vi "Image_RGB888_to_RAW12_U8.vi"(7 "Bayer Pattern":T1, 8 "error in (no error)":errorcluster, 10 "Image Configuration":T2={"Width"=1920, "Height"=1080}, 11 "RGB Frame (U8)":u8[](array[numeric])) -> (0 "error out":errorcluster, 3 "RAW12 Frame (U8)":u8[](array[numeric]))   [LabVIEW 2020]
uses:
  ctl/Image_Configuration.ctl
  ctl/Image_RAW_Bayer_Pattern.ctl
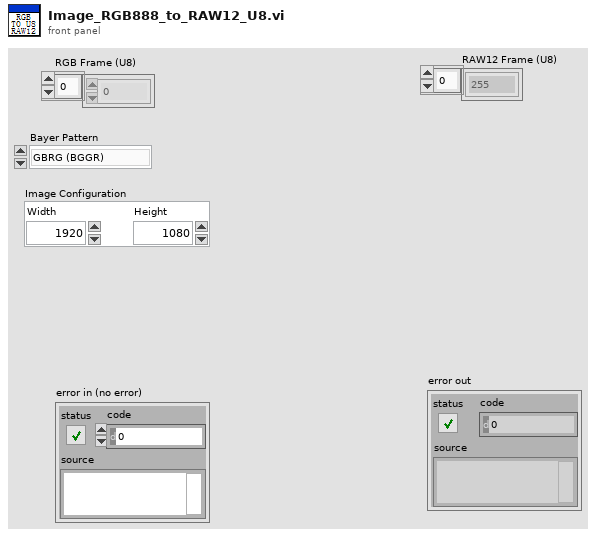
[diagram p1: front panel]
types:
  T1 = typedef "Image_RAW_Bayer_Pattern.ctl" = enum16{"GBRG (BGGR)", "GRBG (RGGB)", "BGGR (GBRG)", "RGGB (GRBG)", "CRBC (RCCB)"}
  T2 = typedef "Image_Configuration.ctl" = cluster{"Width":i32, "Height":i32}
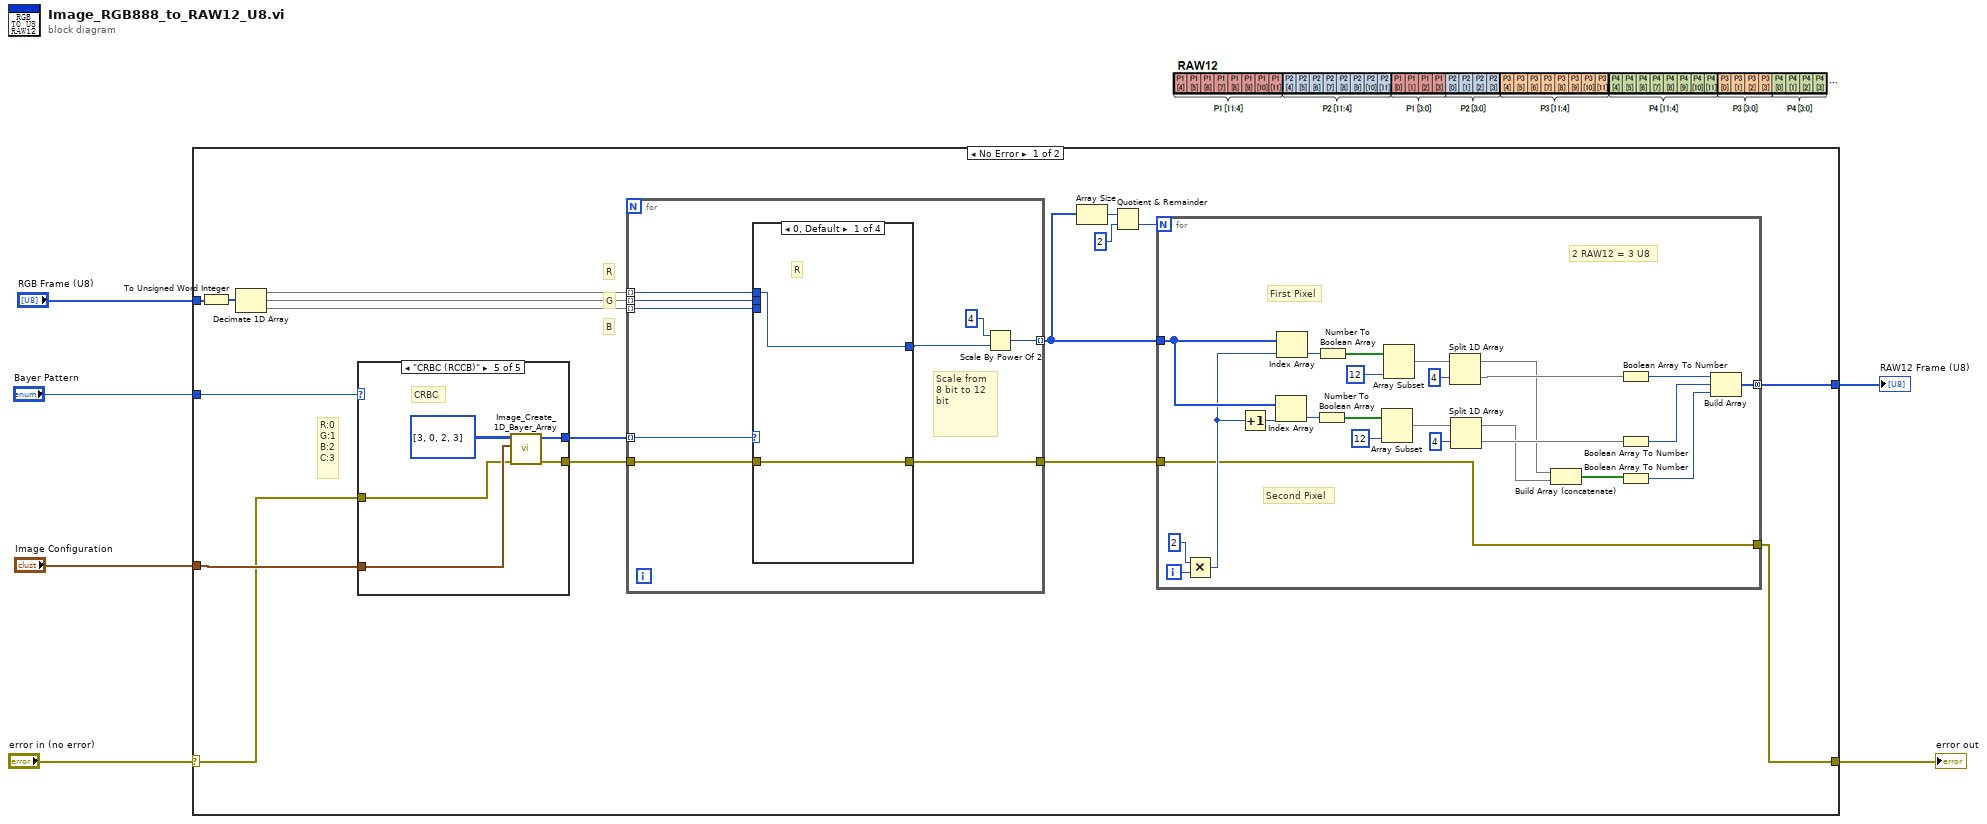
[diagram p0: block diagram]
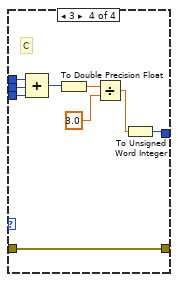
[diagram p4: hidden frame]
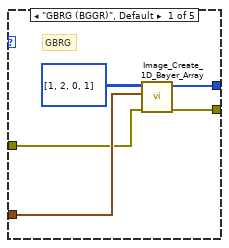
[diagram p5: hidden frame]
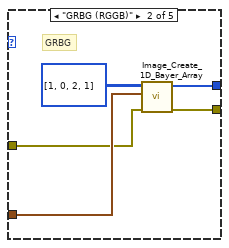
[diagram p6: hidden frame]
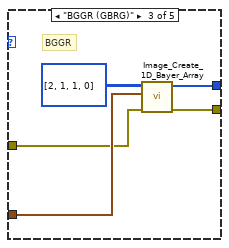
[diagram p7: hidden frame]
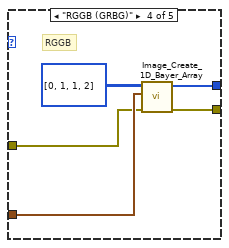
[diagram p8: hidden frame]
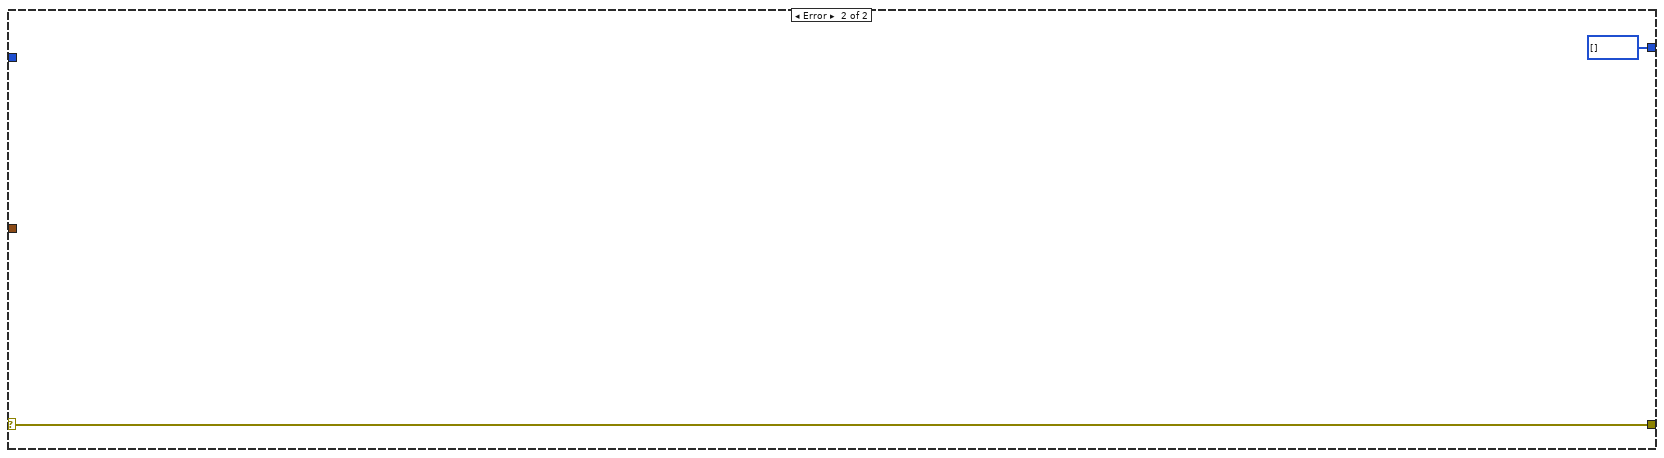
[diagram p9: hidden frame]
diagram:
  n1 = case shown="No Error" "error in (no error)" {
    selector: "error in (no error)" -> [w21 w99]
    tunnel: [w10 w99] -> w5
    tunnel: "RGB Frame (U8)" -> [w8 _]
    tunnel: "Image Configuration" -> [w23 _]
    tunnel: [w12 u8[] []] -> w2
    tunnel: "Bayer Pattern" -> [w9 _]
    frame No Error {
      # "R:0\nG:1\nB:2\nC:3"
      # "B"
      # "G"
      # "R"
      n2 = To Unsigned Word Integer(number=w8) -> (unsigned 16bit integer=w7:u16[])
      n3 = Decimate 1D Array(w7) -> (w19:u16[], w18:u16[], w17:u16[])
      n4 = case shown="\"CRBC (RCCB)\"" w9 {
        tunnel: w23 -> [w76 w81 w86 w91 w94]
        tunnel: [w75 w80 w85 w90 w96] -> w22
        tunnel: w21 -> [w74 w79 w84 w89 w93]
        tunnel: [w73 w78 w83 w88 w95] -> w20
        frame "GBRG (BGGR)", Default {
          # "GBRG"
          n5 = call "Image_Create_1D_Bayer_Array.vi"("error in (no error)"=w74, "Image Configuration"=w76, "Bayer Pattern"=u16[][] [[1, 2], [0, 1]]) -> ("error out"=w73:errorcluster, "Bayer Pattern 1D Array"=w75:u16[])  [unwired: 7 in]
        }
        frame "GRBG (RGGB)" {
          # "GRBG"
          n6 = call "Image_Create_1D_Bayer_Array.vi"("error in (no error)"=w79, "Image Configuration"=w81, "Bayer Pattern"=u16[][] [[1, 0], [2, 1]]) -> ("error out"=w78:errorcluster, "Bayer Pattern 1D Array"=w80:u16[])  [unwired: 7 in]
        }
        frame "BGGR (GBRG)" {
          # "BGGR"
          n7 = call "Image_Create_1D_Bayer_Array.vi"("error in (no error)"=w84, "Image Configuration"=w86, "Bayer Pattern"=u16[][] [[2, 1], [1, 0]]) -> ("error out"=w83:errorcluster, "Bayer Pattern 1D Array"=w85:u16[])  [unwired: 7 in]
        }
        frame "RGGB (GRBG)" {
          # "RGGB"
          n8 = call "Image_Create_1D_Bayer_Array.vi"("error in (no error)"=w89, "Image Configuration"=w91, "Bayer Pattern"=u16[][] [[0, 1], [1, 2]]) -> ("error out"=w88:errorcluster, "Bayer Pattern 1D Array"=w90:u16[])  [unwired: 7 in]
        }
        frame "CRBC (RCCB)" {
          # "CRBC"
          n9 = call "Image_Create_1D_Bayer_Array.vi"("error in (no error)"=w93, "Image Configuration"=w94, "Bayer Pattern"=u16[][] [[3, 0], [2, 3]]) -> ("error out"=w95:errorcluster, "Bayer Pattern 1D Array"=w96:u16[])  [unwired: 7 in]
        }
      }
      n10 = for {
        tunnel: w22 -> [w57] mode=indexing
        tunnel: w20 -> [w55]
        tunnel: w19 -> [w53] mode=indexing
        tunnel: w18 -> [w52] mode=indexing
        tunnel: w17 -> [w51] mode=indexing
        tunnel: [w54] -> w11
        tunnel: [w50] -> w13 mode=indexing
        # "Scale from 8 bit to 12 bit"
        n11 = case shown="0, Default" w57 {
          tunnel: w55 -> [w58 w61 w62 w64]
          tunnel: [w58 w61 w62 w64] -> w54
          tunnel: w53 -> [w59 _ _ w68]
          tunnel: w52 -> [_ w60 _ w67]
          tunnel: w51 -> [_ _ w63 w66]
          tunnel: [w59 w60 w63 w65] -> w49
          frame 0, Default {
            # "R"
          }
          frame 1 {
            # "G"
          }
          frame 2 {
            # "B"
          }
          frame 3 {
            # "C"
            n12 = Compound Arithmetic op=ADD(w68, w67, w66) -> (w70:u16)
            n13 = To Double Precision Float(number=w70) -> (double precision float=w69:dbl)
            n14 = Divide(x=w69, y=3.0) -> (x/y=w71:dbl)
            n15 = To Unsigned Word Integer(number=w71) -> (unsigned 16bit integer=w65:u16)
          }
        }
        n16 = Scale By Power Of 2(n=i16 4, x=w49) -> (x*2^n=w50:u16)
      }
      n17 = Array Size(array=w13) -> (size(s)=w16:i32)
      n18 = Quotient & Remainder(x=w16, y=2) -> (floor(x/y)=w14:i32)  [unwired: 1 out]
      n19 = for {
        N: w14 -> [_]
        tunnel: w13 -> [w48]
        tunnel: [w35] -> w12 mode=concatenating
        tunnel: w11 -> [w34]
        tunnel: [w34] -> w10
        i -> [w47]
        # "2 RAW12 = 3 U8"
        # "Second Pixel"
        # "First Pixel"
        n20 = Multiply(x=2, y=w47) -> (x*y=w45:i32)
        n21 = Increment(x=w45) -> (x+1=w44:i32)
        n22 = Index Array(array=w48, index=w44) -> (element=w42:u16)
        n23 = Index Array(array=w48, index=w45) -> (element=w43:u16)
        n24 = Number To Boolean Array(number=w42) -> (Boolean array=w39:bool[])
        n25 = Number To Boolean Array(number=w43) -> (Boolean array=w38:bool[])
        n26 = Array Subset(array=w39, length=12) -> (w31:bool[])  [unwired: 1 in]
        n27 = Array Subset(array=w38, length=12) -> (w33:bool[])  [unwired: 1 in]
        n28 = Split 1D Array(array=w33, index=4) -> (first subarray=w26:bool[], second subarray=w28:bool[])
        n29 = Split 1D Array(array=w31, index=4) -> (first subarray=w25:bool[], second subarray=w27:bool[])
        n30 = Build Array (concatenate)(w26, w25) -> (w29:bool[])
        n31 = Boolean Array To Number(Boolean array=w28) -> (number=w24:u8)
        n32 = Boolean Array To Number(Boolean array=w27) -> (number=w37:u8)
        n33 = Boolean Array To Number(Boolean array=w29) -> (number=w36:u8)
        n34 = Build Array(w24, w37, w36) -> (w35:u8[])
      }
    }
    frame Error {
    }
  }
  "error out" <- w5
  "RAW12 Frame (U8)" <- w2
